vi "Create Map from Message Indexes to Tx Write Info.vi"(8 "error in":errorcluster, 9 "1553 channel handles":T1[](array[typedef]) {"terminal status channels" format="%.0x"; "error count channel refs"."wrong sync" format="%.0x"; "error count channel refs"."word" format="%.0x"; "error count channel refs"."unconfigured frames" format="%.0x"; "error count channel refs"."parity" format="%.0x"; "error count channel refs"."monitor" format="%.0x"; "error count channel refs"."Manchester" format="%.0x"; "error count channel refs"."improper number of words" format="%.0x"; "error count channel refs"."general protocol" format="%.0x"; "messages"."Rx status handles" format="%.0x"; "messages"."Tx status handles" format="%.0x"; "messages"."timestamps" format="%.0x"; "messages"."parameters"."RxBC channel handle" format="%.0x"; "messages"."parameters"."RxRT channel handle" format="%.0x"; "messages"."parameters"."Tx channel handle" format="%.0x"}, 10 "hardware handles":T6, 11 "1553 channels":T7[](array[typedef])) -> (0 "error out":errorcluster, 3 "map from message indexes to Tx write info":T13)   [LabVIEW 2020, in "Ballard MIL-STD-1553 Engine.lvlib" / "Custom Device.lvlib"]
uses:
  Custom Device.lvlib
  Shared/Map of Message Indexes to Tx Write Info.ctl
  Shared/Tx Write Info.ctl
  Shared/1553 Channel.ctl
  Shared/Address.ctl
  Shared/Message Definition.ctl
  Shared/Message Type.ctl
  Shared/Terminal Endpoint.ctl
  Shared/Parameter Definition.ctl
  Hardware Handles.ctl
  Implementation/Execution Unit/1553 Channel Handles.ctl
  Implementation/Execution Unit/Message Handles.ctl
  Implementation/Execution Unit/Parameter Handles.ctl
  <vilib>/NI VeriStand/Custom Device API/Custom Device Item Ref.ctl
  Shared/Error Count Channel Refs.ctl
  <vilib>/NI VeriStand/Custom Device API/Custom Device API.lvlib
  Implementation/Execution Unit/Execution Unit.lvclass
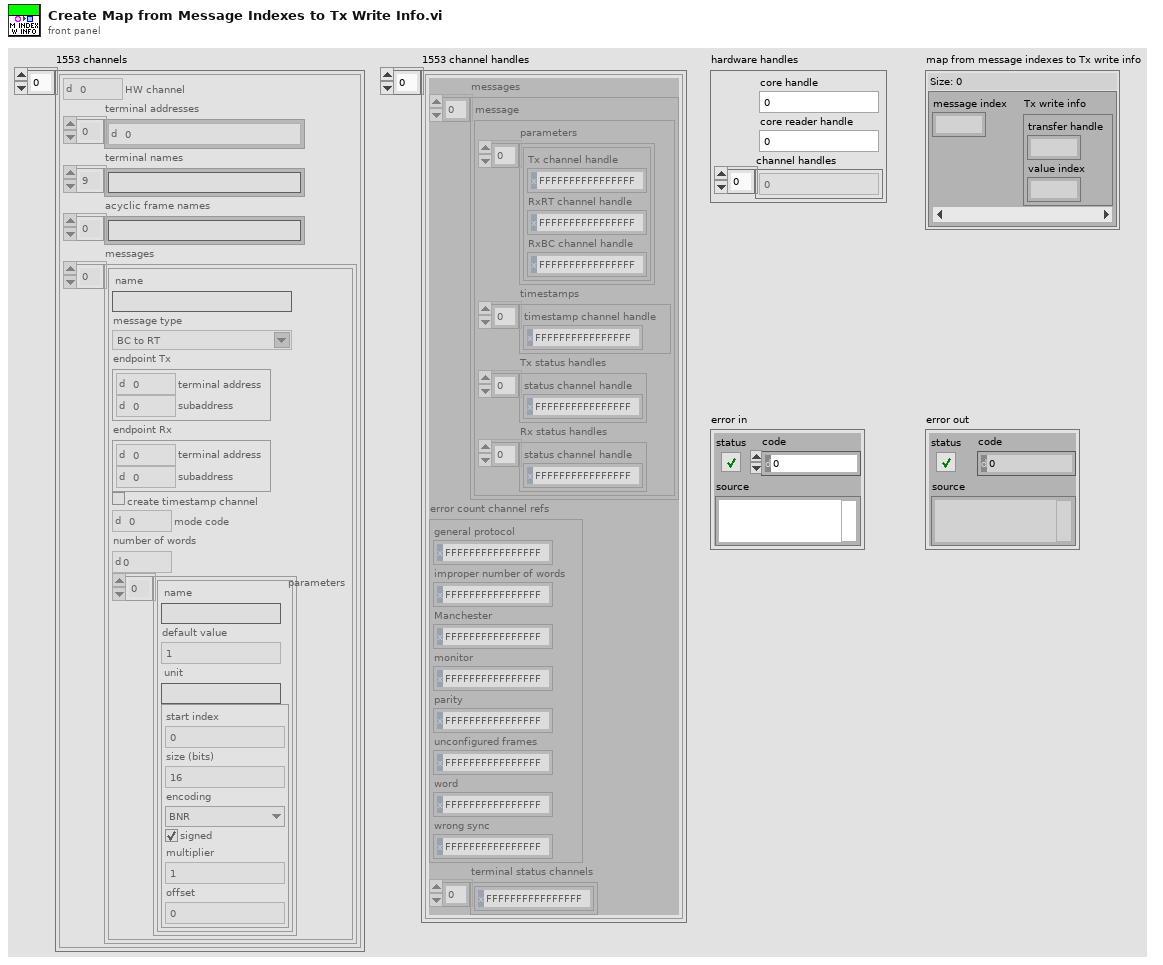
[diagram p1: front panel]
types:
  T1 = typedef "Ballard MIL-STD-1553 Engine.lvlib/Implementation.lvlib/Execution Unit.lvclass/1553 Channel Handles.ctl" = cluster{"messages":T2[], "error count channel refs":T5, "terminal status channels":T4[]}
  T2 = typedef "Ballard MIL-STD-1553 Engine.lvlib/Implementation.lvlib/Execution Unit.lvclass/Message Handles.ctl" = cluster{"parameters":T3[], "timestamps":T4[], "Tx status handles":T4[], "Rx status handles":T4[]}
  T3 = typedef "Ballard MIL-STD-1553 Engine.lvlib/Implementation.lvlib/Execution Unit.lvclass/Parameter Handles.ctl" = cluster{"Tx channel handle":T4, "RxRT channel handle":T4, "RxBC channel handle":T4}
  T4 = typedef "Custom Device API.lvlib/Custom Device Item Ref.ctl" = u64
  T5 = typedef "Error Count Channel Refs.ctl" = cluster{"general protocol":T4, "improper number of words":T4, "Manchester":T4, "monitor":T4, "parity":T4, "unconfigured frames":T4, "word":T4, "wrong sync":T4}
  T6 = typedef "Ballard MIL-STD-1553 Engine.lvlib/Custom Device.lvlib/Hardware Handles.ctl" = cluster{"core handle":u64, "core reader handle":u64, "channel handles":u64[]}
  T7 = typedef "1553 Channel.ctl" = cluster{"HW channel":u16, "terminal addresses":T8[], "terminal names":string[], "acyclic frame names":string[], "messages":T9[]}
  T8 = typedef "Address.ctl" = u16
  T9 = typedef "Message Definition.ctl" = cluster{"name":string, "message type":T10, "endpoint Tx":T11, "endpoint Rx":T11, "create timestamp channel":bool, "mode code":u16, "number of words":u16, "parameters":cluster{"name":string, "default value":dbl, "unit":string, "parameter definition":T12}[]}
  T10 = typedef "Message Type.ctl" = string
  T11 = typedef "Terminal Endpoint.ctl" = cluster{"terminal address":T8, "subaddress":T8}
  T12 = typedef "Parameter Definition.ctl" = cluster{"start index":i32, "size (bits)":i32, "encoding":enum16{"BNR", "BCD", "Discrete"}, "signed":bool, "multiplier":dbl, "offset":dbl}
  T13 = typedef "Map of Message Indexes to Tx Write Info.ctl" = map{i32, T14}
  T14 = typedef "Tx Write Info.ctl" = cluster{"transfer handle":u64, "value index":i32}
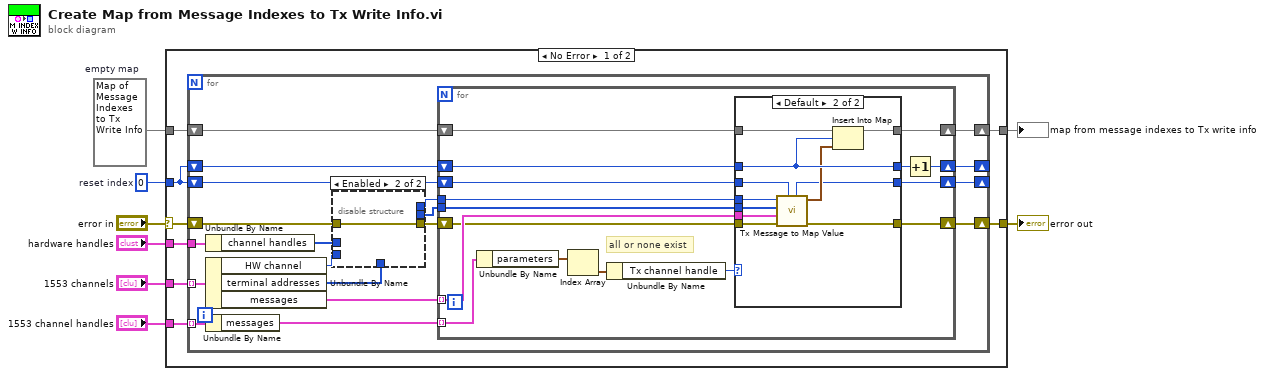
[diagram p0: block diagram]
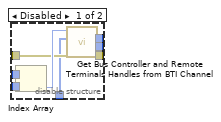
[diagram p2: hidden frame]
diagram:
  w1 = 0  # reset index
  w7 = T13 {}  # empty map
  n1 = case shown="No Error" "error in" {
    selector: "error in" -> [w13 w76]
    tunnel: "1553 channels" -> [w10 _]
    tunnel: [w16 w77] -> w2
    tunnel: w7 -> [w15 w77]
    tunnel: "hardware handles" -> [w14 _]
    tunnel: [w12 w76] -> w4
    tunnel: "1553 channel handles" -> [w11 _]
    tunnel: w1 -> [w9 _]
    frame No Error {
      n2 = for {
        tunnel: w10 -> [w35] mode=indexing
        shift-right: [w32] -> w16
        shift-left: w15 -> [w34]
        shift-right: [w30] -> _
        shift-left: w9 -> [w31]
        tunnel: w14 -> [w29]
        shift-right: [w25] -> w12
        shift-left: w13 -> [w22]
        tunnel: w11 -> [w24] mode=indexing
        shift-right: [w20] -> _
        shift-left: w9 -> [w21]
        n3 = Unbundle By Name(w29) -> ("channel handles"=w28:u64[])
        n4 = Unbundle By Name(w35) -> ("HW channel"=w27:u16, "terminal addresses"=w17:T8[], "messages"=w33:T9[])
        n5 = Unbundle By Name(w24) -> ("messages"=w23:T2[])
        n6 = disable-structure shown="Enabled" {
          disable-tunnel: w28 -> [w43 _]
          disable-tunnel: w27 -> [w42 _]
          disable-tunnel: [w41 w44] -> w26
          disable-tunnel: w22 -> [w39 w44]
          disable-tunnel: [w38 _] -> w19
          disable-tunnel: [w37 _] -> w18
          disable-tunnel: w17 -> [w36 _]
          frame Disabled {
            n7 = Index Array(array=w43, index=w42) -> (element=w40:u64)
            n8 = call "Get Bus Controller and Remote Terminals Handles from BTI Channel.vi"("error in"=w39, "terminal addresses"=w36, "channel handle in"=w40) -> ("error out"=w41:errorcluster, "remote terminal handles out"=w37:u64[], "bus controller handle out"=w38:u64)  [unwired: 5 in, 1 out]
          }
          frame Enabled {
          }
        }
        n9 = for {
          tunnel: w33 -> [w54] mode=indexing
          shift-right: [w60] -> w32
          shift-left: w34 -> [w59]
          shift-right: [w49] -> w30
          shift-left: w31 -> [w58]
          shift-right: [w56] -> w25
          shift-left: w26 -> [w47]
          tunnel: w18 -> [w55]
          tunnel: w23 -> [w53] mode=indexing
          tunnel: w19 -> [w48]
          shift-right: [w45] -> w20
          shift-left: w21 -> [w46]
          # "all or none exist"
          n10 = Unbundle By Name(w53) -> ("parameters"=w52:T3[])
          n11 = Index Array(array=w52) -> (element=w51:T3)  [unwired: 1 in]
          n12 = Unbundle By Name(w51) -> ("Tx channel handle"=w50:T4)
          n13 = case shown="Default" w50 {
            tunnel: [w64 w75] -> w60
            tunnel: w59 -> [w64 w74]
            tunnel: w58 -> [w63 w73]
            tunnel: [w63 w73] -> w57
            tunnel: w47 -> [w62 w72]
            tunnel: [w62 w71] -> w56
            tunnel: w55 -> [_ w68]
            tunnel: w54 -> [_ w69]
            tunnel: w48 -> [_ w67]
            tunnel: w46 -> [w61 w66]
            tunnel: [w61 w65] -> w45
            frame 0, -1 {
              # "Tx channel handle does not exist for this message, so leave out of the map."
            }
            frame Default {
              n14 = call "Tx Message to Map Value.vi"("parameter index"=w66, "error in"=w72, "message"=w69, "remote terminal handles"=w68, "bus controller handle"=w67) -> ("error out"=w71:errorcluster, "Tx write info"=w70:T14, "next parameter index"=w65:i32)  [unwired: 4 in]
              n15 = Insert Into Map(map in=w74, key=w73, value=w70) -> (map out=w75:T13)  [unwired: 2 out]
            }
          }
          n16 = Increment(x=w57) -> (x+1=w49:i32)
        }
      }
    }
    frame Error {
    }
  }
  "map from message indexes to Tx write info" <- w2
  "error out" <- w4
